vi "HAPS_MCU_Init.vi"(5 "array_id":i32, 7 "Tx/Rx":enum16{"Rx", "Tx"}(ring), 8 "error in":errorcluster, 11 "VISA resource name":refnum<visa-resource-name>="COM1") -> (0 "error out":errorcluster)   [LabVIEW 2023, in "HAPS.lvlib"]
uses:
  HAPS.lvlib
  MCU_Function.ctl
  set_ele.ctl
  set_Preamp.ctl
  HAPS_SerialPort.ctl
  HAPS_MCU_ELE_Func.ctl
panel:
  in  "set_Preamp":T1={"ch"=0, "chain_id"=0, "group"=3, "array_id"=0, "ele_phase"=0, "ele_gain"=0, "com_gain"=0, "pd_range"=0}
  in  "set_ele":T2
  in  "Function":T3={"Tx/Rx"=enum."Rx", "Enable?"=enum."On", "Source"=enum."MCU"}
  in  "Serial Settings":T4={"baud rate"=921600, "data bits"=8, "parity"=enum."None", "stop bits"=10, "flow control"=0} {"flow control" items=["None"=0, "XON/XOFF"=1, "RTS/CTS"=2, "DTR/DSR"=4]; "stop bits" items=["1.0"=10, "1.5"=15, "2.0"=20]; "data bits" min=5 max=8 step=1; "baud rate" items=["75"=75, "110"=110, "134"=134, "150"=150, "300"=300, "600"=600, "1200"=1200, "1800"=1800, "2400"=2400, "4800"=4800, "7200"=7200, "9600"=9600, "14400"=14400, "19200"=19200, "28800"=28800, "38400"=38400, "56000"=56000, "57600"=57600, "115200"=115200, "128000"=128000, "230400"=230400, "921600"=921600]}
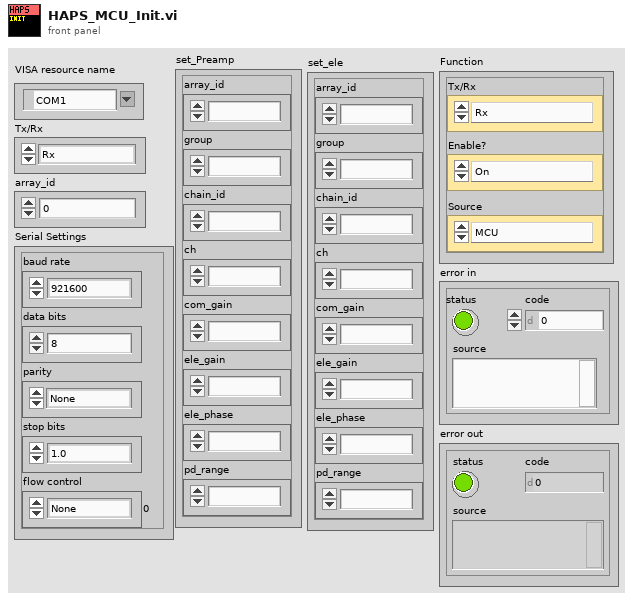
[diagram p1: front panel]
types:
  T1 = typedef "HAPS.lvlib/set_Preamp.ctl" = cluster{"ch":i32, "chain_id":i32, "group":i32, "array_id":i32, "ele_phase":i32, "ele_gain":i32, "com_gain":i32, "pd_range":i32}
  T2 = typedef "HAPS.lvlib/set_ele.ctl" = cluster{"ch":i32, "chain_id":i32, "group":i32, "array_id":i32, "ele_phase":i32, "ele_gain":i32, "com_gain":i32, "pd_range":i32}
  T3 = typedef "HAPS.lvlib/MCU_Function.ctl" = cluster{"Tx/Rx":enum16{"Rx", "Tx"}, "Enable?":enum16{"OFF", "On"}, "Source":enum16{"MCU", "ACU"}}
  T4 = cluster{"baud rate":u32, "data bits":u16, "parity":enum16{"None", "Odd", "Even", "Mark", "Space"}, "stop bits":u16, "flow control":u16}
  T5 = typedef "HAPS.lvlib/HAPS_SerialPort.ctl" = enum16{"Init", "Close", "CMD", "Flush"}
  T6 = typedef "HAPS.lvlib/HAPS_MCU_ELE_Func.ctl" = enum16{"array_init", "set_com_gain", "set_ch_gain_phase", "set_pd_range", "get_preamp_temp", "get_bfic_temp", "get_tx_pd", "ch_on", "ch_on_2", "ch_ctrl_all", "array_ctrl_src"}
  T7 = enum16{"array_init", "set_preamp", "set_com_gain", "set_ch_gain_phase", "set_pd_range", "get_bfic_temp", "get_tx_pd", "ch_on", "ch_ctrl_all", "array_ctrl_src"}
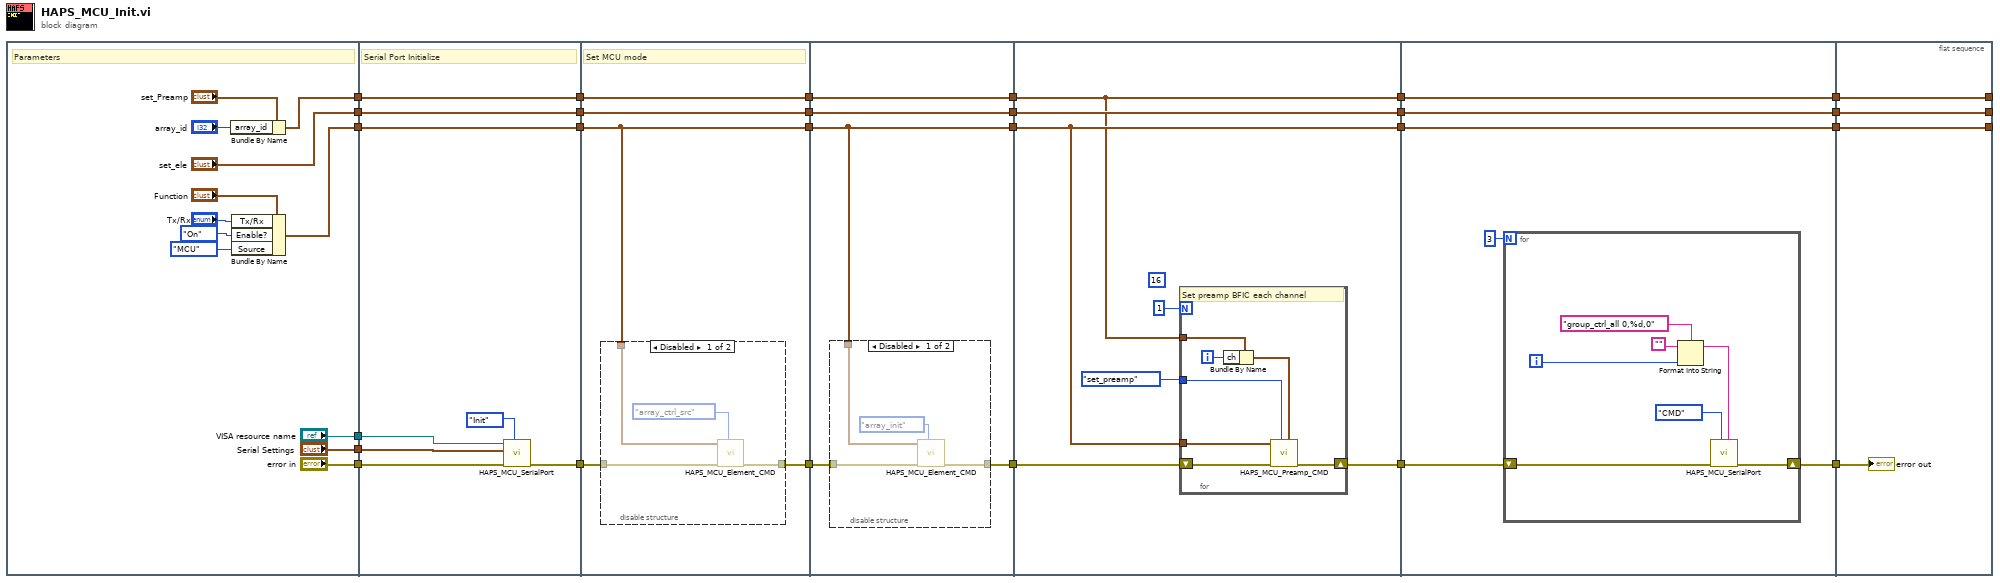
[diagram p0: block diagram]
diagram:
  n1 = flat-sequence {
    tunnel: ["error in"] -> w26
    tunnel: ["Serial Settings"] -> w25
    tunnel: [w27] -> w24
    tunnel: ["set_ele"] -> w23
    tunnel: [w31] -> w22
    tunnel: ["VISA resource name"] -> w9
    tunnel: w26 -> [w42]
    tunnel: w25 -> [w40]
    tunnel: w24 -> [w46]
    tunnel: w23 -> [w45]
    tunnel: w22 -> [w44]
    tunnel: [w43] -> w21
    tunnel: [w46] -> w20
    tunnel: [w45] -> w19
    tunnel: [w44] -> w18
    tunnel: w9 -> [w39]
    tunnel: w21 -> [w49]
    tunnel: w20 -> [w51]
    tunnel: w19 -> [w48]
    tunnel: w18 -> [w47]
    tunnel: [w50] -> w17
    tunnel: [w51] -> w16
    tunnel: [w48] -> w15
    tunnel: [w47] -> w14
    tunnel: w17 -> [w58]
    tunnel: w16 -> [w61]
    tunnel: w15 -> [w60]
    tunnel: w14 -> [w57]
    tunnel: [w59] -> w13
    tunnel: [w61] -> w12
    tunnel: [w60] -> w11
    tunnel: [w57] -> w10
    tunnel: w13 -> [w70]
    tunnel: w12 -> [w67]
    tunnel: w11 -> [w73]
    tunnel: w10 -> [w69]
    tunnel: [w71] -> w8
    tunnel: [w67] -> w6
    tunnel: [w73] -> w4
    tunnel: [w69] -> w2
    tunnel: w8 -> [w83]
    tunnel: [w82] -> w7
    tunnel: w6 -> [w86]
    tunnel: [w86] -> w5
    tunnel: w4 -> [w84]
    tunnel: [w84] -> w3
    tunnel: w2 -> [w85]
    tunnel: [w85] -> w1
    tunnel: [w95] -> _
    tunnel: [w96] -> _
    tunnel: [w97] -> _
    tunnel: w7 -> [w94]
    tunnel: w5 -> [w97]
    tunnel: w3 -> [w96]
    tunnel: w1 -> [w95]
    frame #0 {
      # "Parameters"
      n2 = Bundle By Name(cluster="set_Preamp", "array_id"="array_id") -> (w27:T1)
      n3 = Bundle By Name(cluster="Function", "Tx/Rx"="Tx/Rx", "Enable?"=enum16{"OFF", "On"}."On", "Source"=enum16{"MCU", "ACU"}."MCU") -> (w31:T3)
    }
    frame #1 {
      # "Serial Port Initialize"
      n4 = call "HAPS_MCU_SerialPort.vi"("HAPS_SerialPort_Func"=HAPS_SerialPort."Init", "error in"=w42, "Serial Settings"=w40, "VISA resource name"=w39) -> ("error out"=w43:errorcluster)  [unwired: 5 in, 2 out]
    }
    frame #2 {
      # "Set MCU mode"
      n5 = disable-structure shown="Disabled" {
        disable-tunnel: [w55 w56] -> w50
        disable-tunnel: w49 -> [w54 w56]
        disable-tunnel: w47 -> [w52 _]
        frame Disabled {
          n6 = call "HAPS_MCU_Element_CMD.vi"("HAPS_MCU_ELE_Func."=HAPS_MCU_ELE_Func."array_ctrl_src", "error in"=w54, "Function"=w52) -> ("error out"=w55:errorcluster)  [unwired: 7 in, 1 out]
        }
        frame Enabled {
        }
      }
    }
    frame #3 {
      n7 = disable-structure shown="Disabled" {
        disable-tunnel: [w65 w66] -> w59
        disable-tunnel: w58 -> [w64 w66]
        disable-tunnel: w57 -> [w62 _]
        frame Disabled {
          n8 = call "HAPS_MCU_Element_CMD.vi"("HAPS_MCU_ELE_Func."=HAPS_MCU_ELE_Func."array_init", "error in"=w64, "Function"=w62) -> ("error out"=w65:errorcluster)  [unwired: 7 in, 1 out]
        }
        frame Enabled {
        }
      }
    }
    frame #4 {
      (unwired) 16
      n9 = for {
        N: 1 -> [_]
        tunnel: T7."set_preamp" ("HAPS_MCU_CMD") -> [w78]
        tunnel: w67 -> [w76]
        tunnel: w69 -> [w77]
        shift-right: [w79] -> w71
        shift-left: w70 -> [w80]
        i -> [w74]
        # "Set preamp BFIC each channel"
        n10 = Bundle By Name(cluster=w76, "ch"=w74) -> (w75:T1)
        n11 = call "HAPS_MCU_Preamp_CMD.vi"("set_Preamp"=w75, "HAPS_MCU_Preamp_Func."=w78, "error in"=w80, "Function"=w77) -> ("error out"=w79:errorcluster)  [unwired: 6 in, 1 out]
      }
    }
    frame #5 {
      n12 = for {
        N: 3 -> [_]
        shift-right: [w88] -> w82
        shift-left: w83 -> [w89]
        i -> [w87]
        n13 = Format Into String(format string="group_ctrl_all 0,%d,0" ("Command"), initial string="", w87) -> (resulting string=w90:string)  [unwired: 1 in, 1 out]
        n14 = call "HAPS_MCU_SerialPort.vi"("Command"=w90, "HAPS_SerialPort_Func"=enum16{"Init", "Close", "CMD"}."CMD" ("HAPS_SerialPort"), "error in"=w89) -> ("error out"=w88:errorcluster)  [unwired: 6 in, 2 out]
      }
    }
    frame #6 {
      "error out" <- w94
    }
  }
